vi "sigma of n^2.vi"() -> ()   [LabVIEW 2018]
panel:
  out "sigma n**2":dbl
  in  "n":dbl
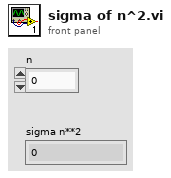
[diagram p1: front panel]
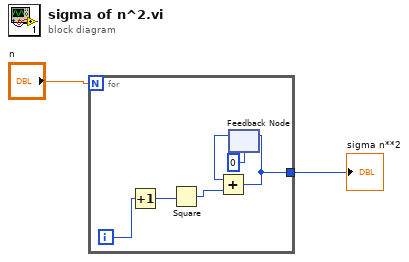
[diagram p0: block diagram]
diagram:
  n1 = for {
    N: "n" -> [_]
    tunnel: [w3] -> w2
    i -> [w8]
    n2 = Increment(x=w8) -> (x+1=w7:i32)
    n3 = Square(x=w7) -> (x^2=w6:i32)
    n4 = feedback #1(0) -> (w5:i32)
    n5 = Add(x=w5, y=w6) -> (x+y=w3:i32)
    n6 = feedback-in #1(w3) -> ()
  }
  "sigma n**2" <- w2
